vi "CRYUpdate DataView Toolbar.vi"(10 "nData":i32, 11 "pVI":refnum<vi>) -> ()   [LabVIEW 2013]
uses:
  Control/CRYData View Toolbar.ctl
panel:
  in  "Boolean Ref":refnum<vi>
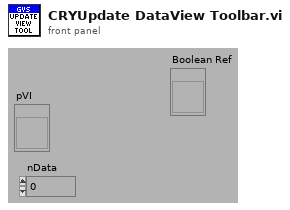
[diagram p1: front panel]
types:
  T1 = enum8{"Enabled", "Disabled", "Disabled and Grayed Out"}
  T2 = typedef "CRYData View Toolbar.ctl" = cluster{"TitleShowOnOff":refnum<vi>, "LegendShowOnOff":refnum<vi>, "CursorShowOnOff":refnum<vi>, "PreviewShowOnOff":refnum<vi>, "X_Autoscale":refnum<vi>, "Y1_Autoscale":refnum<vi>, "Y2_Autoscale":refnum<vi>}
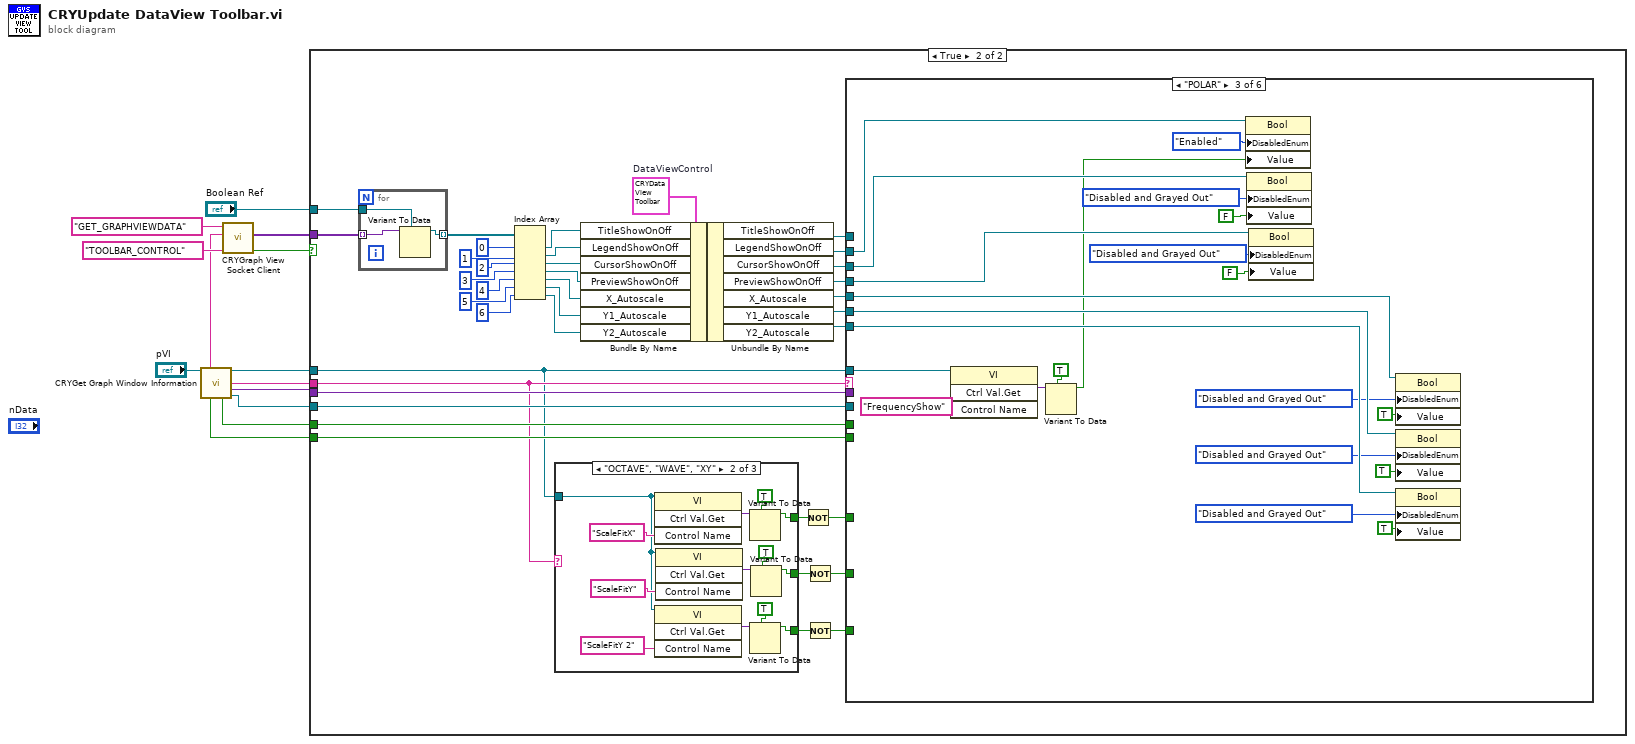
[diagram p0: block diagram]
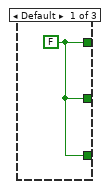
[diagram p3: hidden frame]
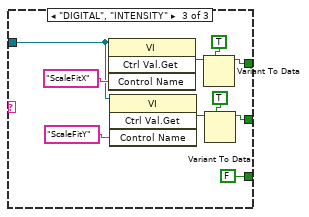
[diagram p4: hidden frame]
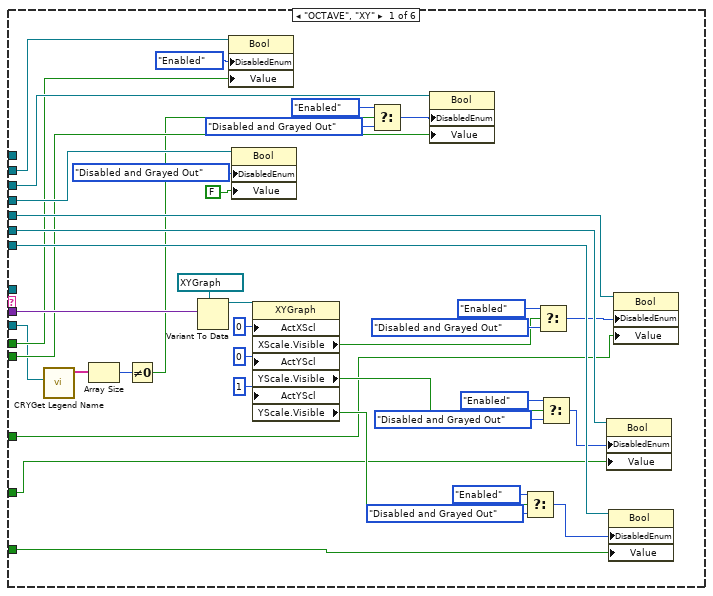
[diagram p5: hidden frame]
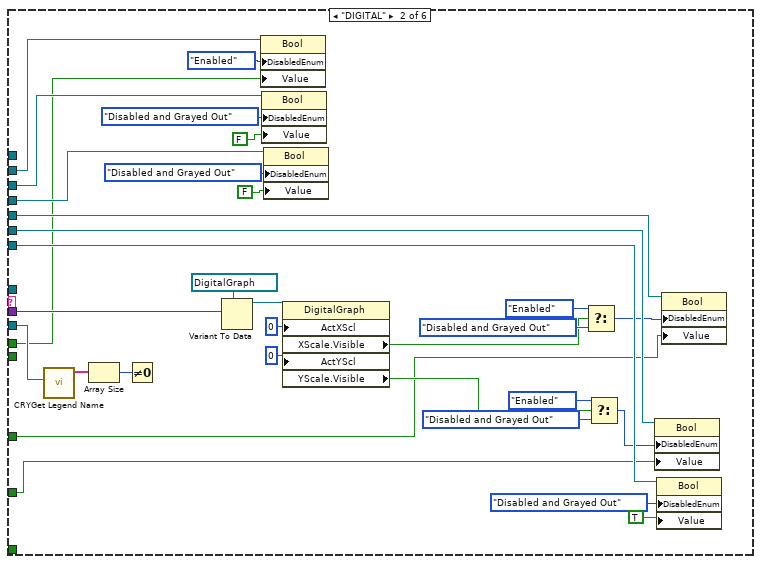
[diagram p6: hidden frame]
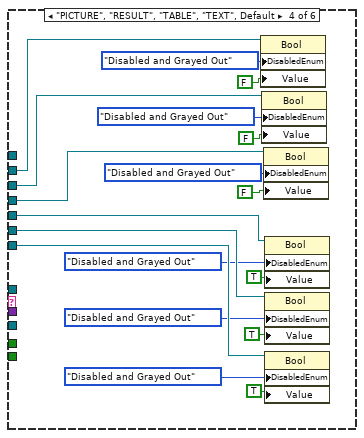
[diagram p7: hidden frame]
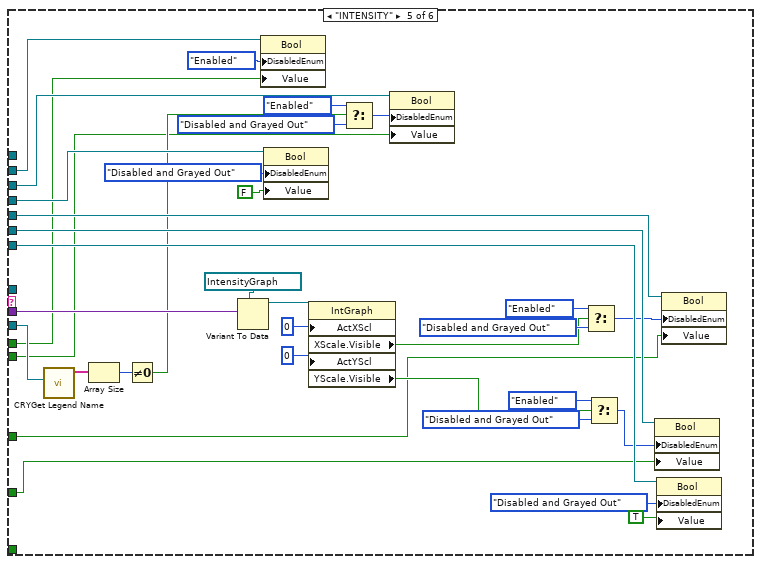
[diagram p8: hidden frame]
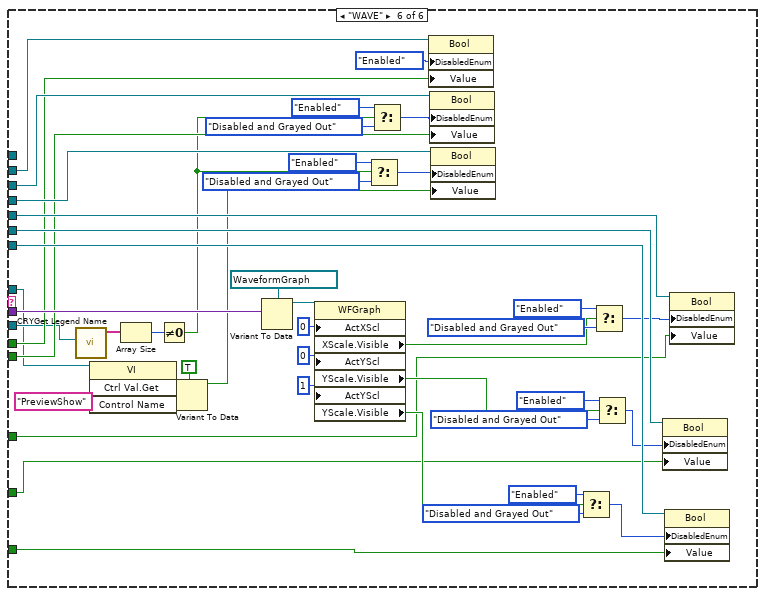
[diagram p9: hidden frame]
diagram:
  n1 = call "CRYGet Graph Window Information.vi"("pGraph VI In"="pVI") -> ("Queue Name Out"=w8:string, "pGraph VI Out"=w1:refnum<vi>, "Graph Type Out"=w7:string, "Graph Control Ref Out"=w6:variant, "CursorShow Out"=w4:bool, "LegendShow Out"=w5:bool, "Legend Ref Out"=w2:refnum<vi>)  [unwired: 4 in, 4 out]
  n2 = call "CRYGraph View Socket Client.vi"("sOption"="TOOLBAR_CONTROL", "sData"=w8, "sAction"="GET_GRAPHVIEWDATA") -> ("bResult Out"=w3:bool, "Variant Out"=w10:variant[])  [unwired: 5 in, 2 out]
  n3 = case shown="True" w3 {
    tunnel: "Boolean Ref" -> [_ w51]
    tunnel: w10 -> [_ w41]
    tunnel: w7 -> [_ w21]
    tunnel: w6 -> [_ w40]
    tunnel: w5 -> [_ w24]
    tunnel: w4 -> [_ w23]
    tunnel: w2 -> [_ w22]
    tunnel: w1 -> [_ w20]
    frame False {
    }
    frame True {
      w50 = T2 {"TitleShowOnOff"=refnum, "LegendShowOnOff"=refnum, "CursorShowOnOff"=refnum, "PreviewShowOnOff"=refnum, "X_Autoscale"=refnum, "Y1_Autoscale"=refnum, "Y2_Autoscale"=refnum}  # DataViewControl
      n4 = for {
        tunnel: w41 -> [w268] mode=indexing
        tunnel: w51 -> [w269]
        tunnel: [w267] -> w49 mode=indexing
        n5 = Variant To Data(type=w269, Variant=w268) -> (data=w267:refnum<vi>)  [unwired: 1 in, 1 out]
      }
      n6 = Index Array(array=w49, index #1=0 ("index"), index #2=1 ("index"), index #3=2 ("index"), index #4=3 ("index"), index #5=4 ("index"), index #6=5 ("index"), index #7=6 ("index")) -> (element #1=w48:refnum<vi>, element #2=w47:refnum<vi>, element #3=w46:refnum<vi>, element #4=w45:refnum<vi>, element #5=w44:refnum<vi>, element #6=w43:refnum<vi>, element #7=w42:refnum<vi>)
      n7 = case shown="\"OCTAVE\", \"WAVE\", \"XY\"" w21 {
        tunnel: w20 -> [_ w56 w69]
        tunnel: [w52 w55 w68] -> w19
        tunnel: [w52 w54 w67] -> w18
        tunnel: [w52 w53 FALSE] -> w17
        frame Default {
          w52 = FALSE
        }
        frame "OCTAVE", "WAVE", "XY" {
          n8 = invoke class="VI" method="Ctrl Val.Get"(reference=w56, "Control Name"="ScaleFitX") -> ("Get Control Value Variant"=w64:variant)  [unwired: 2 in, 3 out]
          n9 = invoke class="VI" method="Ctrl Val.Get"(reference=w56, "Control Name"="ScaleFitY 2") -> ("Get Control Value Variant"=w58:variant)  [unwired: 2 in, 3 out]
          n10 = invoke class="VI" method="Ctrl Val.Get"(reference=w56, "Control Name"="ScaleFitY") -> ("Get Control Value Variant"=w61:variant)  [unwired: 2 in, 3 out]
          n11 = Variant To Data(type=TRUE, Variant=w64) -> (data=w55:bool)  [unwired: 1 in, 1 out]
          n12 = Variant To Data(type=TRUE, Variant=w58) -> (data=w53:bool)  [unwired: 1 in, 1 out]
          n13 = Variant To Data(type=TRUE, Variant=w61) -> (data=w54:bool)  [unwired: 1 in, 1 out]
        }
        frame "DIGITAL", "INTENSITY" {
          n14 = invoke class="VI" method="Ctrl Val.Get"(reference=w69, "Control Name"="ScaleFitX") -> ("Get Control Value Variant"=w74:variant)  [unwired: 2 in, 3 out]
          n15 = invoke class="VI" method="Ctrl Val.Get"(reference=w69, "Control Name"="ScaleFitY") -> ("Get Control Value Variant"=w71:variant)  [unwired: 2 in, 3 out]
          n16 = Variant To Data(type=TRUE, Variant=w74) -> (data=w68:bool)  [unwired: 1 in, 1 out]
          n17 = Variant To Data(type=TRUE, Variant=w71) -> (data=w67:bool)  [unwired: 1 in, 1 out]
        }
      }
      n18 = Bundle By Name(cluster=w50, "TitleShowOnOff"=w48, "LegendShowOnOff"=w47, "CursorShowOnOff"=w46, "PreviewShowOnOff"=w45, "X_Autoscale"=w44, "Y1_Autoscale"=w43, "Y2_Autoscale"=w42) -> (w39:T2)
      n19 = Unbundle By Name(w39) -> ("TitleShowOnOff"=w38:refnum<vi>, "LegendShowOnOff"=w37:refnum<vi>, "CursorShowOnOff"=w36:refnum<vi>, "PreviewShowOnOff"=w35:refnum<vi>, "X_Autoscale"=w34:refnum<vi>, "Y1_Autoscale"=w33:refnum<vi>, "Y2_Autoscale"=w32:refnum<vi>)
      n20 = Not(x=w19) -> (.not. x?=w16:bool)
      n21 = Not(x=w18) -> (.not. x?=w15:bool)
      n22 = Not(x=w17) -> (.not. x?=w14:bool)
      n23 = case shown="\"POLAR\"" w21 {
        tunnel: w40 -> [w113 w146 _ _ w221 w266]
        tunnel: w38 -> [_ _ _ _ _ _]
        tunnel: w37 -> [w96 w134 w160 w178 w209 w251]
        tunnel: w36 -> [w97 w135 w161 w179 w210 w252]
        tunnel: w35 -> [w99 w137 w163 w181 w212 w254]
        tunnel: w34 -> [w108 w142 w168 w186 w217 w261]
        tunnel: w33 -> [w103 w141 w167 w185 w216 w256]
        tunnel: w32 -> [w102 w140 w166 w184 w215 w255]
        tunnel: w24 -> [w87 w122 _ _ w197 w242]
        tunnel: w23 -> [w86 _ _ _ w192 w241]
        tunnel: w22 -> [w83 w123 _ _ w198 w238]
        tunnel: w20 -> [_ _ w148 _ _ w232]
        tunnel: w16 -> [w78 w118 _ _ w188 w224]
        tunnel: w15 -> [w77 w117 _ _ w187 w223]
        tunnel: w14 -> [w76 _ _ _ _ w222]
        frame "OCTAVE", "XY" {
          n24 = call "CRYGet Legend Name.vi"("MCListbox Refnum"=w83) -> ("Names Out"=w85:string[])  [unwired: 10 in]
          n25 = Array Size(array=w85) -> (size(s)=w84:i32)
          n26 = Not Equal To 0?(x=w84) -> (x != 0?=w79:bool)
          n27 = Variant To Data(type=refnum<vi> refnum ("XY Graph"), Variant=w113) -> (data=w112:refnum<vi>)  [unwired: 1 in, 1 out]
          n28 = property class="Bool"(reference=w96, "DisabledEnum"=T1."Enabled" ("Disabled"), "Value"=w87) -> ()  [unwired: 1 in, 2 out]
          n29 = property class="Bool"(reference=w99, "DisabledEnum"=T1."Disabled and Grayed Out" ("Disabled"), "Value"=FALSE) -> ()  [unwired: 1 in, 2 out]
          n30 = property class="XYGraph"(reference=w112, "ActXScl"=0 ("Active X Scale"), "ActYScl"=0 ("Active Y Scale"), "ActYScl"=1 ("Active Y Scale")) -> ("XScale.Visible"=w92:bool, "YScale.Visible"=w89:bool, "YScale.Visible"=w107:bool)  [unwired: 1 in, 2 out]
          n31 = Select(t=T1."Enabled" ("Disabled"), s=w79, f=T1."Disabled and Grayed Out" ("Disabled")) -> (s? t:f=w81:T1)
          n32 = property class="Bool"(reference=w97, "DisabledEnum"=w81, "Value"=w86) -> ()  [unwired: 1 in, 2 out]
          n33 = Select(t=T1."Enabled" ("Disabled"), s=w107, f=T1."Disabled and Grayed Out" ("Disabled")) -> (s? t:f=w104:T1)
          n34 = Select(t=T1."Enabled" ("Disabled"), s=w92, f=T1."Disabled and Grayed Out" ("Disabled")) -> (s? t:f=w93:T1)
          n35 = Select(t=T1."Enabled" ("Disabled"), s=w89, f=T1."Disabled and Grayed Out" ("Disabled")) -> (s? t:f=w88:T1)
          n36 = property class="Bool"(reference=w103, "DisabledEnum"=w88, "Value"=w77) -> ()  [unwired: 1 in, 2 out]
          n37 = property class="Bool"(reference=w102, "DisabledEnum"=w104, "Value"=w76) -> ()  [unwired: 1 in, 2 out]
          n38 = property class="Bool"(reference=w108, "DisabledEnum"=w93, "Value"=w78) -> ()  [unwired: 1 in, 2 out]
        }
        frame "DIGITAL" {
          n39 = call "CRYGet Legend Name.vi"("MCListbox Refnum"=w123) -> ("Names Out"=w125:string[])  [unwired: 10 in]
          n40 = Array Size(array=w125) -> (size(s)=w124:i32)
          n41 = Not Equal To 0?(x=w124) -> ()  [unwired: 1 out]
          n42 = Variant To Data(type=refnum<vi> refnum ("Graph Ref"), Variant=w146) -> (data=w145:refnum<vi>)  [unwired: 1 in, 1 out]
          n43 = property class="Bool"(reference=w134, "DisabledEnum"=T1."Enabled" ("Disabled"), "Value"=w122) -> ()  [unwired: 1 in, 2 out]
          n44 = property class="Bool"(reference=w135, "DisabledEnum"=T1."Disabled and Grayed Out" ("Disabled"), "Value"=FALSE) -> ()  [unwired: 1 in, 2 out]
          n45 = property class="Bool"(reference=w137, "DisabledEnum"=T1."Disabled and Grayed Out" ("Disabled"), "Value"=FALSE) -> ()  [unwired: 1 in, 2 out]
          n46 = property class="DigitalGraph"(reference=w145, "ActXScl"=0 ("Active X Scale"), "ActYScl"=0 ("Active Y Scale")) -> ("XScale.Visible"=w130:bool, "YScale.Visible"=w127:bool)  [unwired: 1 in, 2 out]
          n47 = Select(t=T1."Enabled" ("Disabled"), s=w130, f=T1."Disabled and Grayed Out" ("Disabled")) -> (s? t:f=w131:T1)
          n48 = Select(t=T1."Enabled" ("Disabled"), s=w127, f=T1."Disabled and Grayed Out" ("Disabled")) -> (s? t:f=w126:T1)
          n49 = property class="Bool"(reference=w141, "DisabledEnum"=w126, "Value"=w117) -> ()  [unwired: 1 in, 2 out]
          n50 = property class="Bool"(reference=w140, "DisabledEnum"=T1."Disabled and Grayed Out" ("Disabled"), "Value"=TRUE) -> ()  [unwired: 1 in, 2 out]
          n51 = property class="Bool"(reference=w142, "DisabledEnum"=w131, "Value"=w118) -> ()  [unwired: 1 in, 2 out]
        }
        frame "POLAR" {
          n52 = invoke class="VI" method="Ctrl Val.Get"(reference=w148, "Control Name"="FrequencyShow") -> ("Get Control Value Variant"=w150:variant)  [unwired: 2 in, 3 out]
          n53 = Variant To Data(type=TRUE, Variant=w150) -> (data=w147:bool)  [unwired: 1 in, 1 out]
          n54 = property class="Bool"(reference=w160, "DisabledEnum"=T1."Enabled" ("Disabled"), "Value"=w147) -> ()  [unwired: 1 in, 2 out]
          n55 = property class="Bool"(reference=w161, "DisabledEnum"=T1."Disabled and Grayed Out" ("Disabled"), "Value"=FALSE) -> ()  [unwired: 1 in, 2 out]
          n56 = property class="Bool"(reference=w163, "DisabledEnum"=T1."Disabled and Grayed Out" ("Disabled"), "Value"=FALSE) -> ()  [unwired: 1 in, 2 out]
          n57 = property class="Bool"(reference=w168, "DisabledEnum"=T1."Disabled and Grayed Out" ("Disabled"), "Value"=TRUE) -> ()  [unwired: 1 in, 2 out]
          n58 = property class="Bool"(reference=w167, "DisabledEnum"=T1."Disabled and Grayed Out" ("Disabled"), "Value"=TRUE) -> ()  [unwired: 1 in, 2 out]
          n59 = property class="Bool"(reference=w166, "DisabledEnum"=T1."Disabled and Grayed Out" ("Disabled"), "Value"=TRUE) -> ()  [unwired: 1 in, 2 out]
        }
        frame "PICTURE", "RESULT", "TABLE", "TEXT", Default {
          n60 = property class="Bool"(reference=w178, "DisabledEnum"=T1."Disabled and Grayed Out" ("Disabled"), "Value"=FALSE) -> ()  [unwired: 1 in, 2 out]
          n61 = property class="Bool"(reference=w179, "DisabledEnum"=T1."Disabled and Grayed Out" ("Disabled"), "Value"=FALSE) -> ()  [unwired: 1 in, 2 out]
          n62 = property class="Bool"(reference=w181, "DisabledEnum"=T1."Disabled and Grayed Out" ("Disabled"), "Value"=FALSE) -> ()  [unwired: 1 in, 2 out]
          n63 = property class="Bool"(reference=w186, "DisabledEnum"=T1."Disabled and Grayed Out" ("Disabled"), "Value"=TRUE) -> ()  [unwired: 1 in, 2 out]
          n64 = property class="Bool"(reference=w185, "DisabledEnum"=T1."Disabled and Grayed Out" ("Disabled"), "Value"=TRUE) -> ()  [unwired: 1 in, 2 out]
          n65 = property class="Bool"(reference=w184, "DisabledEnum"=T1."Disabled and Grayed Out" ("Disabled"), "Value"=TRUE) -> ()  [unwired: 1 in, 2 out]
        }
        frame "INTENSITY" {
          n66 = call "CRYGet Legend Name.vi"("MCListbox Refnum"=w198) -> ("Names Out"=w200:string[])  [unwired: 10 in]
          n67 = Array Size(array=w200) -> (size(s)=w199:i32)
          n68 = Not Equal To 0?(x=w199) -> (x != 0?=w193:bool)
          n69 = Variant To Data(type=refnum<vi> refnum ("Graph Ref"), Variant=w221) -> (data=w220:refnum<vi>)  [unwired: 1 in, 1 out]
          n70 = property class="Bool"(reference=w209, "DisabledEnum"=T1."Enabled" ("Disabled"), "Value"=w197) -> ()  [unwired: 1 in, 2 out]
          n71 = property class="Bool"(reference=w212, "DisabledEnum"=T1."Disabled and Grayed Out" ("Disabled"), "Value"=FALSE) -> ()  [unwired: 1 in, 2 out]
          n72 = property class="IntGraph"(reference=w220, "ActXScl"=0 ("Active X Scale"), "ActYScl"=0 ("Active Y Scale")) -> ("XScale.Visible"=w205:bool, "YScale.Visible"=w202:bool)  [unwired: 1 in, 2 out]
          n73 = Select(t=T1."Enabled" ("Disabled"), s=w193, f=T1."Disabled and Grayed Out" ("Disabled")) -> (s? t:f=w194:T1)
          n74 = property class="Bool"(reference=w210, "DisabledEnum"=w194, "Value"=w192) -> ()  [unwired: 1 in, 2 out]
          n75 = Select(t=T1."Enabled" ("Disabled"), s=w205, f=T1."Disabled and Grayed Out" ("Disabled")) -> (s? t:f=w206:T1)
          n76 = Select(t=T1."Enabled" ("Disabled"), s=w202, f=T1."Disabled and Grayed Out" ("Disabled")) -> (s? t:f=w201:T1)
          n77 = property class="Bool"(reference=w216, "DisabledEnum"=w201, "Value"=w187) -> ()  [unwired: 1 in, 2 out]
          n78 = property class="Bool"(reference=w215, "DisabledEnum"=T1."Disabled and Grayed Out" ("Disabled"), "Value"=TRUE) -> ()  [unwired: 1 in, 2 out]
          n79 = property class="Bool"(reference=w217, "DisabledEnum"=w206, "Value"=w188) -> ()  [unwired: 1 in, 2 out]
        }
        frame "WAVE" {
          n80 = call "CRYGet Legend Name.vi"("MCListbox Refnum"=w238) -> ("Names Out"=w240:string[])  [unwired: 10 in]
          n81 = invoke class="VI" method="Ctrl Val.Get"(reference=w232, "Control Name"="PreviewShow") -> ("Get Control Value Variant"=w234:variant)  [unwired: 2 in, 3 out]
          n82 = Array Size(array=w240) -> (size(s)=w239:i32)
          n83 = Not Equal To 0?(x=w239) -> (x != 0?=w226:bool)
          n84 = Variant To Data(type=TRUE ("x != 0?"), Variant=w234) -> (data=w230:bool)  [unwired: 1 in, 1 out]
          n85 = Variant To Data(type=refnum<vi> refnum ("WaveGraph Ref"), Variant=w266) -> (data=w265:refnum<vi>)  [unwired: 1 in, 1 out]
          n86 = property class="WFGraph"(reference=w265, "ActXScl"=0 ("Active X Scale"), "ActYScl"=0 ("Active Y Scale"), "ActYScl"=1 ("Active Y Scale")) -> ("XScale.Visible"=w247:bool, "YScale.Visible"=w244:bool, "YScale.Visible"=w260:bool)  [unwired: 1 in, 2 out]
          n87 = Select(t=T1."Enabled" ("Disabled"), s=w226, f=T1."Disabled and Grayed Out" ("Disabled")) -> (s? t:f=w227:T1)
          n88 = Select(t=T1."Enabled" ("Disabled"), s=w226, f=T1."Disabled and Grayed Out" ("Disabled")) -> (s? t:f=w236:T1)
          n89 = property class="Bool"(reference=w251, "DisabledEnum"=T1."Enabled" ("Disabled"), "Value"=w242) -> ()  [unwired: 1 in, 2 out]
          n90 = property class="Bool"(reference=w252, "DisabledEnum"=w236, "Value"=w241) -> ()  [unwired: 1 in, 2 out]
          n91 = property class="Bool"(reference=w254, "DisabledEnum"=w227, "Value"=w230) -> ()  [unwired: 1 in, 2 out]
          n92 = Select(t=T1."Enabled" ("Disabled"), s=w260, f=T1."Disabled and Grayed Out" ("Disabled")) -> (s? t:f=w257:T1)
          n93 = Select(t=T1."Enabled" ("Disabled"), s=w247, f=T1."Disabled and Grayed Out" ("Disabled")) -> (s? t:f=w248:T1)
          n94 = Select(t=T1."Enabled" ("Disabled"), s=w244, f=T1."Disabled and Grayed Out" ("Disabled")) -> (s? t:f=w243:T1)
          n95 = property class="Bool"(reference=w256, "DisabledEnum"=w243, "Value"=w223) -> ()  [unwired: 1 in, 2 out]
          n96 = property class="Bool"(reference=w255, "DisabledEnum"=w257, "Value"=w222) -> ()  [unwired: 1 in, 2 out]
          n97 = property class="Bool"(reference=w261, "DisabledEnum"=w248, "Value"=w224) -> ()  [unwired: 1 in, 2 out]
        }
      }
    }
  }
